vi "Launch Nested Actors.vi"(8 "Error In":errorcluster, 10 "Nested Actors":T1, 11 "LHW-GUI-Actor in":refnum<class "LHW-GUI-Actor.lvclass">) -> (0 "Error Out":errorcluster, 3 "LHW-GUI-Actor out":refnum<class "LHW-GUI-Actor.lvclass">)   [LabVIEW 2014, in "LHW-GUI.lvlib" / "LHW-GUI-Actor.lvclass"]
doc: "Launch nested actors."
uses:
  LHW-GUI-Actor.lvclass
  LHW-Acquisition/LHW-Aquisition-Actor.lvclass
  LHW-Analysis/LHW-Analysis-Actor.lvclass
  LHW-Storage/LHW-Storage-Actor.lvclass
  LHW-GUI-Actor.lvclass/LHW-GUI-Actor.ctl
  <vilib>/ActorFramework/Actor/Actor.lvclass
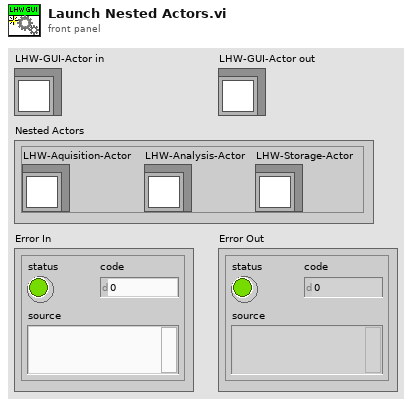
[diagram p1: front panel]
types:
  T1 = cluster{"LHW-Aquisition-Actor":refnum<class "LHW-Aquisition-Actor.lvclass">, "LHW-Analysis-Actor":refnum<class "LHW-Analysis-Actor.lvclass">, "LHW-Storage-Actor":refnum<class "LHW-Storage-Actor.lvclass">}
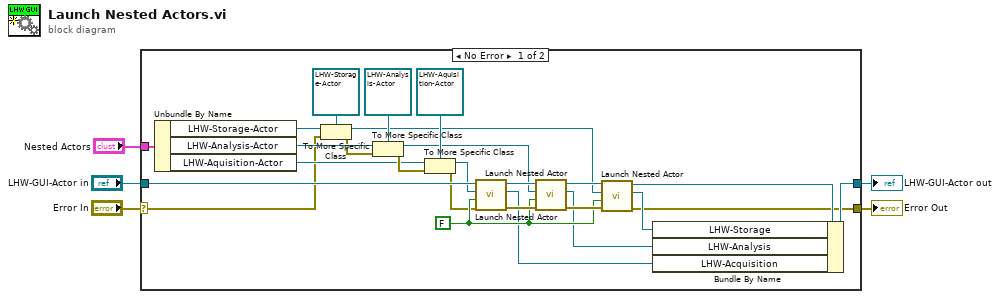
[diagram p0: block diagram]
diagram:
  n1 = case shown="No Error" "Error In" {
    selector: "Error In" -> [w9 w33]
    tunnel: [w20 w33] -> w4
    tunnel: [w21 w32] -> w2
    tunnel: "LHW-GUI-Actor in" -> [w31 w32]
    tunnel: "Nested Actors" -> [w19 _]
    frame No Error {
      w26 = FALSE ("Auto-stop? (T)")
      n2 = Unbundle By Name(w19) -> ("LHW-Storage-Actor"=w18:refnum<class "LHW-Storage-Actor.lvclass">, "LHW-Analysis-Actor"=w15:refnum<class "LHW-Analysis-Actor.lvclass">, "LHW-Aquisition-Actor"=w12:refnum<class "LHW-Aquisition-Actor.lvclass">)
      n3 = To More Specific Class(target class=refnum<class "LHW-Storage-Actor.lvclass"> refnum ("LHW-Storage.lvlib:LHW-Storage-Actor.lvclass"), reference=w18, error in=w9) -> (specific class reference=w6:refnum<class "LHW-Storage-Actor.lvclass">, error out=w14:errorcluster)
      n4 = To More Specific Class(target class=refnum<class "LHW-Analysis-Actor.lvclass"> refnum ("LHW-Analysis.lvlib:LHW-Analysis-Actor.lvclass"), reference=w15, error in=w14) -> (specific class reference=w7:refnum<class "LHW-Analysis-Actor.lvclass">, error out=w13:errorcluster)
      n5 = To More Specific Class(target class=refnum<class "LHW-Aquisition-Actor.lvclass"> refnum ("LHW-Acquisition.lvlib:LHW-Aquisition-Actor.lvclass"), reference=w12, error in=w13) -> (specific class reference=w10:refnum<class "LHW-Aquisition-Actor.lvclass">, error out=w8:errorcluster)
      n6 = call <vilib>:"Launch Nested Actor.vi"("error in (no error)"=w8, "Auto-stop? (T)"=w26, "Nested Actor"=w10, "Caller Actor in"=w31) -> ("error out"=w27:errorcluster, "Nested Actor's Enqueuer"=w22:refnum<class "Message Enqueuer.lvclass">, "Caller Actor out"=w28:refnum<class "LHW-GUI-Actor.lvclass">)  [unwired: 5 in]
      n7 = call <vilib>:"Launch Nested Actor.vi"("error in (no error)"=w27, "Auto-stop? (T)"=w26, "Nested Actor"=w7, "Caller Actor in"=w28) -> ("error out"=w30:errorcluster, "Nested Actor's Enqueuer"=w23:refnum<class "Message Enqueuer.lvclass">, "Caller Actor out"=w29:refnum<class "LHW-GUI-Actor.lvclass">)  [unwired: 5 in]
      n8 = call <vilib>:"Launch Nested Actor.vi"("error in (no error)"=w30, "Auto-stop? (T)"=w26, "Nested Actor"=w6, "Caller Actor in"=w29) -> ("error out"=w20:errorcluster, "Nested Actor's Enqueuer"=w24:refnum<class "Message Enqueuer.lvclass">, "Caller Actor out"=w25:refnum<class "LHW-GUI-Actor.lvclass">)  [unwired: 5 in]
      n9 = Bundle By Name(cluster=w25, "LHW-Storage"=w24, "LHW-Analysis"=w23, "LHW-Acquisition"=w22) -> (w21:refnum<class "LHW-GUI-Actor.lvclass">)
    }
    frame Error {
    }
  }
  "Error Out" <- w4
  "LHW-GUI-Actor out" <- w2
